vi "Export File - Tx Packet XML.vi"(4 "Tx Packet":T1 {"threadOptions"."pclDecimation" max=16 step=1; "threadOptions"."loopPeriod" max=16 step=1; "threadOptions"."targetPriority" min=-2 max=16 step=1; "threadOptions"."targetProcessor" min=-2 max=16 step=1; "Endianness" items=["big-endian"=0, "little-endian"=2]}, 6 "RootNode":refnum<k24>, 8 "error in (no error)":errorcluster, 9 "Tx Packet Header Data":T13, 11 "XmlDocument in":refnum<k24>) -> (0 "error out":errorcluster, 3 "XmlDocument out":refnum<k24>)   [LabVIEW 2019, in "UDP-Custom-Device System Explorer.lvlib"]
uses:
  UDP-Custom-Device System Explorer.lvlib
  System.Xml
  Types/XML - New/ImpExp - Packet Headers.ctl
  Types/XML - New/ImpExp - Tx Packet Data.ctl
  <vilib>/NI VeriStand/Custom Device API/Custom Device Item Info.ctl
  Shared/Types/Shared - Channel Data Type.ctl
  Shared/Types/Shared - Buffered.PacketInfo.ctl
  Shared/Types/Shared - Pointer Encoding.ctl
  Shared/Types/Shared - Receive Buffer Options.ctl
  Shared/Types/Shared - Transmit Buffer Options.ctl
  Shared/Types/Shared - Transmit Flag Options.ctl
  Shared/Types/Shared - Transmit Echo Options.ctl
  Types/Threading/Thread Configuration.ctl
  Types/Threading/Thread Sync Reference.ctl
  Shared/Types/Shared - Thread Management.ctl
  Shared/UDP-Custom-Device Shared.lvlib
  <vilib>/NI VeriStand/Custom Device API/Custom Device API.lvlib
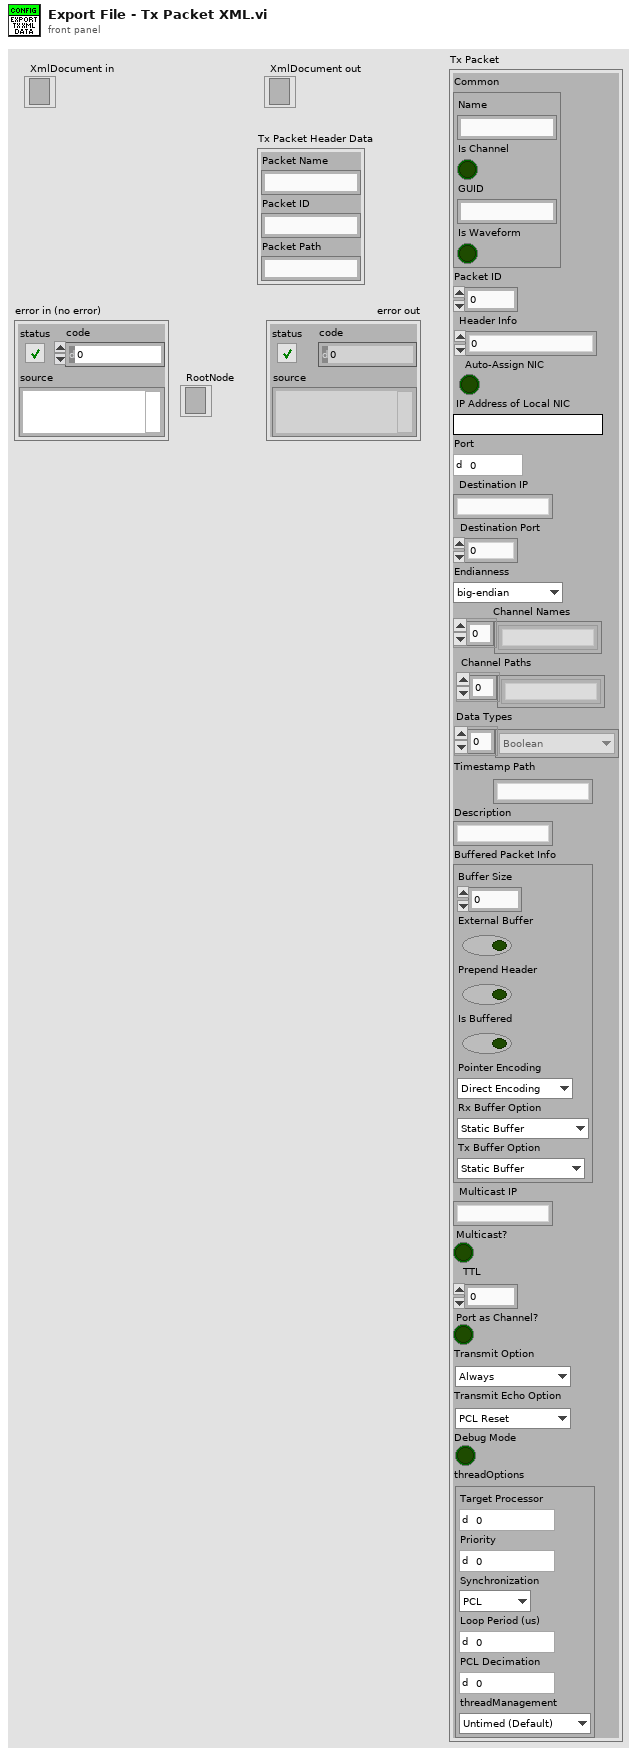
[diagram p1: front panel]
types:
  T1 = typedef "UDP-Custom-Device System Explorer.lvlib/ImpExp - Tx Packet Data.ctl" = cluster{"Common":T2, "Packet ID":i32, "Header Info":u32, "Auto-Assign NIC":bool, "IP Address of Local NIC":string, "Port":u16, "Destination IP":string, "Destination Port":u16, "Endianness":u16, "Channel Names":string[], "Channel Paths":string[], "Data Types":T3[], "Timestamp Path":string, "Description":string, "Buffered Packet Info":T4, "Multicast IP":string, "Multicast?":bool, "TTL":u16, "Port as Channel?":bool, "Transmit Option":T8, "Transmit Echo Option":T9, "Debug Mode":bool, "threadOptions":T10}
  T2 = typedef "Custom Device API.lvlib/Custom Device Item Info.ctl" = cluster{"Name":string, "Is Channel":bool, "GUID":string, "Is Waveform":bool}
  T3 = typedef "UDP-Custom-Device Shared.lvlib/Shared - Channel Data Type.ctl" = enum16{"Boolean", "Single", "Double", "I8", "I16", "I32", "I64", "U8", "U16", "U32", "U64"}
  T4 = typedef "UDP-Custom-Device Shared.lvlib/Shared - Buffered.PacketInfo.ctl" = cluster{"Buffer Size":i32, "External Buffer":bool, "Prepend Header":bool, "Is Buffered":bool, "Pointer Encoding":T5, "Rx Buffer Option":T6, "Tx Buffer Option":T7}
  T5 = typedef "UDP-Custom-Device Shared.lvlib/Shared - Pointer Encoding.ctl" = enum16{"Direct Encoding", "Conversion Encoding"}
  T6 = typedef "UDP-Custom-Device Shared.lvlib/Shared - Receive Buffer Options.ctl" = enum16{"Static Buffer", "Circular Buffer", "Circular Buffer + Size", "Internal Cache", "Internal Cache + Size", "Ping Pong", "Ping Pong + Size"}
  T7 = typedef "UDP-Custom-Device Shared.lvlib/Shared - Transmit Buffer Options.ctl" = enum16{"Static Buffer", "FIFO Buffer", "FIFO Buffer + Port"}
  T8 = typedef "UDP-Custom-Device Shared.lvlib/Shared - Transmit Flag Options.ctl" = enum16{"Always", "One-Shot", "Toggle"}
  T9 = typedef "UDP-Custom-Device Shared.lvlib/Shared - Transmit Echo Options.ctl" = enum16{"PCL Reset", "Counter", "Mirror"}
  T10 = typedef "UDP-Custom-Device System Explorer.lvlib/Thread Configuration.ctl" = cluster{"targetProcessor":i8, "targetPriority":i16, "Synchronization":T11, "loopPeriod":u32, "pclDecimation":u16, "threadManagement":T12}
  T11 = typedef "UDP-Custom-Device System Explorer.lvlib/Thread Sync Reference.ctl" = enum16{"PCL", "Async"}
  T12 = typedef "UDP-Custom-Device Shared.lvlib/Shared - Thread Management.ctl" = enum16{"Untimed (Default)", "Timed (High Priority)"}
  T13 = typedef "UDP-Custom-Device System Explorer.lvlib/ImpExp - Packet Headers.ctl" = cluster{"Packet Name":string, "Packet ID":string, "Packet Path":string}
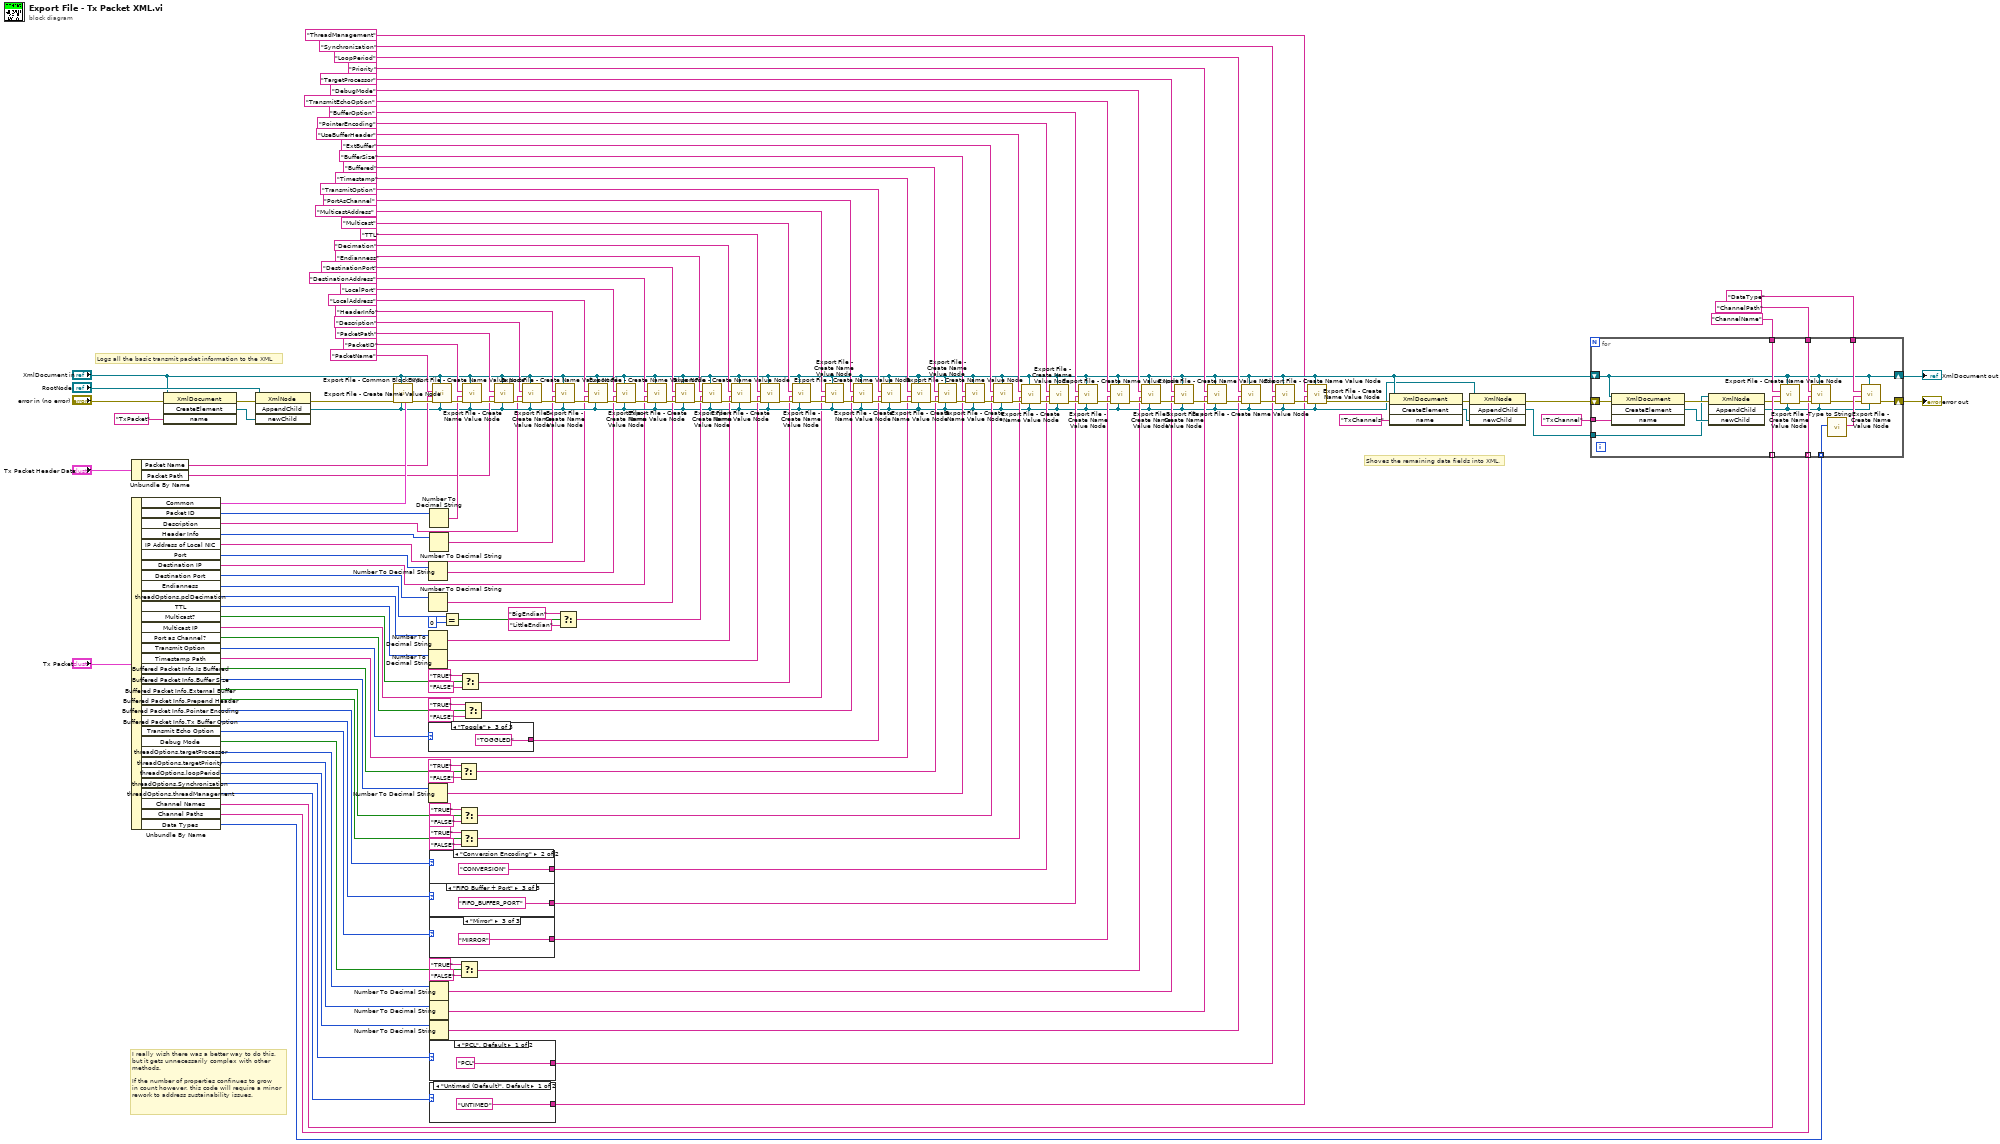
[diagram p0: block diagram]
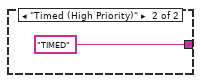
[diagram p2: hidden frame]
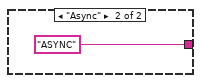
[diagram p3: hidden frame]
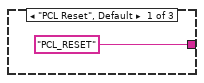
[diagram p4: hidden frame]
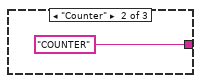
[diagram p5: hidden frame]
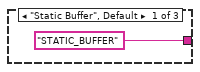
[diagram p6: hidden frame]
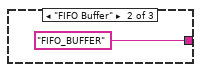
[diagram p7: hidden frame]
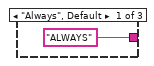
[diagram p8: hidden frame]
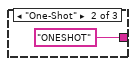
[diagram p9: hidden frame]
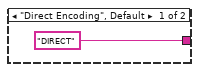
[diagram p10: hidden frame]
diagram:
  # "I really wish there was a better way to do this,\nbut it gets unnecessarily complex with other\nmethods.\n\nIf the number of properties confinues to grow\nin count however, this code will require a minor\nrework to address sustainability issues."
  # "Shoves the remaining data fields into XML."
  # "Logs all the basic transmit packet information to the XML"
  n1 = Unbundle By Name("Tx Packet") -> ("Common"=w149:T2, "Packet ID"=w140:i32, "Description"=w25:string, "Header Info"=w115:u32, "IP Address of Local NIC"=w24:string, "Port"=w112:u16, "Destination IP"=w23:string, "Destination Port"=w110:u16, "Endianness"=w103:u16, "threadOptions.pclDecimation"=w108:u16, "TTL"=w22:u16, "Multicast?"=w21:bool, "Multicast IP"=w20:string, "Port as Channel?"=w19:bool, "Transmit Option"=w18:T8, "Timestamp Path"=w17:string, "Buffered Packet Info.Is Buffered"=w16:bool, "Buffered Packet Info.Buffer Size"=w15:i32, "Buffered Packet Info.External Buffer"=w14:bool, "Buffered Packet Info.Prepend Header"=w13:bool, "Buffered Packet Info.Pointer Encoding"=w12:T5, "Buffered Packet Info.Tx Buffer Option"=w11:T7, "Transmit Echo Option"=w10:T9, "Debug Mode"=w9:bool, "threadOptions.targetProcessor"=w8:i8, "threadOptions.targetPriority"=w7:i16, "threadOptions.loopPeriod"=w6:u32, "threadOptions.Synchronization"=w5:T11, "threadOptions.threadManagement"=w4:T12, "Channel Names"=w3:string[], "Channel Paths"=w2:string[], "Data Types"=w1:T3[])
  n2 = Unbundle By Name("Tx Packet Header Data") -> ("Packet Name"=w139:string, "Packet Path"=w137:string)
  n3 = invoke class="XmlDocument" method="CreateElement"(reference="XmlDocument in", error in="error in (no error)", "name"="TxPacket" ("Tag Name")) -> (error out=w153:errorcluster, "CreateElement"=w154:refnum<k24>)  [unwired: 1 in, 2 out]
  n4 = invoke class="XmlNode" method="AppendChild"(reference="RootNode", error in=w153, "newChild"=w154) -> (error out=w152:errorcluster, "AppendChild"=w28:refnum<k24>)  [unwired: 1 in, 2 out]
  n5 = call "Export File - Common Block XML.vi"("Common"=w149, "RootNode in"=w28, "XmlDocument in"="XmlDocument in", "error in (no error)"=w152) -> ("error out"=w142:errorcluster)  [unwired: 7 in]
  n6 = Number To Decimal String(number=w112) -> (decimal integer string=w111:string)  [unwired: 1 in]
  n7 = Number To Decimal String(number=w110) -> (decimal integer string=w109:string)  [unwired: 1 in]
  n8 = Number To Decimal String(number=w108) -> (decimal integer string=w107:string)  [unwired: 1 in]
  n9 = Number To Decimal String(number=w22) -> (decimal integer string=w68:string)  [unwired: 1 in]
  n10 = case shown="\"Toggle\"" w18 {
    tunnel: ["ALWAYS" "ONESHOT" "TOGGLED"] -> w55
    frame "Always", Default {
    }
    frame "One-Shot" {
    }
    frame "Toggle" {
    }
  }
  n11 = Number To Decimal String(number=w15) -> (decimal integer string=w94:string)  [unwired: 1 in]
  n12 = Number To Decimal String(number=w140) -> (decimal integer string=w138:string)  [unwired: 1 in]
  n13 = Number To Decimal String(number=w115) -> (decimal integer string=w114:string)  [unwired: 1 in]
  n14 = case shown="\"Conversion Encoding\"" w12 {
    tunnel: ["DIRECT" "CONVERSION"] -> w64
    frame "Direct Encoding", Default {
    }
    frame "Conversion Encoding" {
    }
  }
  n15 = case shown="\"FIFO Buffer + Port\"" w11 {
    tunnel: ["STATIC_BUFFER" "FIFO_BUFFER" "FIFO_BUFFER_PORT"] -> w52
    frame "Static Buffer", Default {
    }
    frame "FIFO Buffer" {
    }
    frame "FIFO Buffer + Port" {
    }
  }
  n16 = case shown="\"Mirror\"" w10 {
    tunnel: ["PCL_RESET" "COUNTER" "MIRROR"] -> w49
    frame "PCL Reset", Default {
    }
    frame "Counter" {
    }
    frame "Mirror" {
    }
  }
  n17 = Number To Decimal String(number=w8) -> (decimal integer string=w35:string)  [unwired: 1 in]
  n18 = Number To Decimal String(number=w7) -> (decimal integer string=w34:string)  [unwired: 1 in]
  n19 = Number To Decimal String(number=w6) -> (decimal integer string=w33:string)  [unwired: 1 in]
  n20 = case shown="\"PCL\", Default" w5 {
    tunnel: ["PCL" "ASYNC"] -> w32
    frame "PCL", Default {
    }
    frame "Async" {
    }
  }
  n21 = case shown="\"Untimed (Default)\", Default" w4 {
    tunnel: ["UNTIMED" "TIMED"] -> w26
    frame "Untimed (Default)", Default {
    }
    frame "Timed (High Priority)" {
    }
  }
  n22 = call "Export File - Create Name Value Node.vi"("RootNode in"=w28, "XmlDocument in"="XmlDocument in", "error in (no error)"=w142, "Value"=w139, "Name"="PacketName" ("Tag Name")) -> ("error out"=w147:errorcluster)  [unwired: 6 in]
  n23 = Equal?(x=w103, y=u16 0) -> (x = y?=w102:bool)
  n24 = Select(t="TRUE", s=w16, f="FALSE") -> (s? t:f=w96:string)
  n25 = Select(t="TRUE", s=w14, f="FALSE") -> (s? t:f=w89:string)
  n26 = Select(t="TRUE", s=w13, f="FALSE") -> (s? t:f=w88:string)
  n27 = Select(t="TRUE", s=w9, f="FALSE") -> (s? t:f=w44:string)
  n28 = Select(t="TRUE", s=w21, f="FALSE") -> (s? t:f=w69:string)
  n29 = call "Export File - Create Name Value Node.vi"("RootNode in"=w28, "XmlDocument in"="XmlDocument in", "error in (no error)"=w147, "Value"=w138, "Name"="PacketID" ("Tag Name")) -> ("error out"=w146:errorcluster)  [unwired: 6 in]
  n30 = Select(t="TRUE", s=w19, f="FALSE") -> (s? t:f=w59:string)
  n31 = call "Export File - Create Name Value Node.vi"("RootNode in"=w28, "XmlDocument in"="XmlDocument in", "error in (no error)"=w146, "Value"=w137, "Name"="PacketPath" ("Tag Name")) -> ("error out"=w130:errorcluster)  [unwired: 6 in]
  n32 = call "Export File - Create Name Value Node.vi"("RootNode in"=w28, "XmlDocument in"="XmlDocument in", "error in (no error)"=w130, "Value"=w25, "Name"="Description" ("Tag Name")) -> ("error out"=w136:errorcluster)  [unwired: 6 in]
  n33 = call "Export File - Create Name Value Node.vi"("RootNode in"=w28, "XmlDocument in"="XmlDocument in", "error in (no error)"=w136, "Value"=w114, "Name"="HeaderInfo" ("Tag Name")) -> ("error out"=w113:errorcluster)  [unwired: 6 in]
  n34 = Select(t="BigEndian", s=w102, f="LittleEndian") -> (s? t:f=w101:string)
  n35 = call "Export File - Create Name Value Node.vi"("RootNode in"=w28, "XmlDocument in"="XmlDocument in", "error in (no error)"=w113, "Value"=w24, "Name"="LocalAddress" ("Tag Name")) -> ("error out"=w135:errorcluster)  [unwired: 6 in]
  n36 = call "Export File - Create Name Value Node.vi"("RootNode in"=w28, "XmlDocument in"="XmlDocument in", "error in (no error)"=w135, "Value"=w111, "Name"="LocalPort" ("Tag Name")) -> ("error out"=w134:errorcluster)  [unwired: 6 in]
  n37 = call "Export File - Create Name Value Node.vi"("RootNode in"=w28, "XmlDocument in"="XmlDocument in", "error in (no error)"=w134, "Value"=w23, "Name"="DestinationAddress" ("Tag Name")) -> ("error out"=w133:errorcluster)  [unwired: 6 in]
  n38 = call "Export File - Create Name Value Node.vi"("RootNode in"=w28, "XmlDocument in"="XmlDocument in", "error in (no error)"=w133, "Value"=w109, "Name"="DestinationPort" ("Tag Name")) -> ("error out"=w132:errorcluster)  [unwired: 6 in]
  n39 = call "Export File - Create Name Value Node.vi"("RootNode in"=w28, "XmlDocument in"="XmlDocument in", "error in (no error)"=w132, "Value"=w101, "Name"="Endianness" ("Tag Name")) -> ("error out"=w131:errorcluster)  [unwired: 6 in]
  n40 = call "Export File - Create Name Value Node.vi"("RootNode in"=w28, "XmlDocument in"="XmlDocument in", "error in (no error)"=w131, "Value"=w107, "Name"="Decimation" ("Tag Name")) -> ("error out"=w74:errorcluster)  [unwired: 6 in]
  n41 = call "Export File - Create Name Value Node.vi"("RootNode in"=w28, "XmlDocument in"="XmlDocument in", "error in (no error)"=w74, "Value"=w68, "Name"="TTL" ("Tag Name")) -> ("error out"=w76:errorcluster)  [unwired: 6 in]
  n42 = call "Export File - Create Name Value Node.vi"("RootNode in"=w28, "XmlDocument in"="XmlDocument in", "error in (no error)"=w76, "Value"=w69, "Name"="Multicast" ("Tag Name")) -> ("error out"=w75:errorcluster)  [unwired: 6 in]
  n43 = call "Export File - Create Name Value Node.vi"("RootNode in"=w28, "XmlDocument in"="XmlDocument in", "error in (no error)"=w75, "Value"=w20, "Name"="MulticastAddress" ("Tag Name")) -> ("error out"=w63:errorcluster)  [unwired: 6 in]
  n44 = call "Export File - Create Name Value Node.vi"("RootNode in"=w28, "XmlDocument in"="XmlDocument in", "error in (no error)"=w63, "Value"=w59, "Name"="PortAsChannel" ("Tag Name")) -> ("error out"=w58:errorcluster)  [unwired: 6 in]
  n45 = call "Export File - Create Name Value Node.vi"("RootNode in"=w28, "XmlDocument in"="XmlDocument in", "error in (no error)"=w58, "Value"=w55, "Name"="TransmitOption" ("Tag Name")) -> ("error out"=w57:errorcluster)  [unwired: 6 in]
  n46 = call "Export File - Create Name Value Node.vi"("RootNode in"=w28, "XmlDocument in"="XmlDocument in", "error in (no error)"=w57, "Value"=w17, "Name"="Timestamp" ("Tag Name")) -> ("error out"=w98:errorcluster)  [unwired: 6 in]
  n47 = call "Export File - Create Name Value Node.vi"("RootNode in"=w28, "XmlDocument in"="XmlDocument in", "error in (no error)"=w98, "Value"=w96, "Name"="Buffered" ("Tag Name")) -> ("error out"=w97:errorcluster)  [unwired: 6 in]
  n48 = call "Export File - Create Name Value Node.vi"("RootNode in"=w28, "XmlDocument in"="XmlDocument in", "error in (no error)"=w97, "Value"=w94, "Name"="BufferSize" ("Tag Name")) -> ("error out"=w119:errorcluster)  [unwired: 6 in]
  n49 = call "Export File - Create Name Value Node.vi"("RootNode in"=w28, "XmlDocument in"="XmlDocument in", "error in (no error)"=w119, "Value"=w89, "Name"="ExtBuffer" ("Tag Name")) -> ("error out"=w118:errorcluster)  [unwired: 6 in]
  n50 = call "Export File - Create Name Value Node.vi"("RootNode in"=w28, "XmlDocument in"="XmlDocument in", "error in (no error)"=w118, "Value"=w88, "Name"="UseBufferHeader" ("Tag Name")) -> ("error out"=w66:errorcluster)  [unwired: 6 in]
  n51 = call "Export File - Create Name Value Node.vi"("RootNode in"=w28, "XmlDocument in"="XmlDocument in", "error in (no error)"=w66, "Value"=w64, "Name"="PointerEncoding" ("Tag Name")) -> ("error out"=w54:errorcluster)  [unwired: 6 in]
  n52 = call "Export File - Create Name Value Node.vi"("RootNode in"=w28, "XmlDocument in"="XmlDocument in", "error in (no error)"=w54, "Value"=w52, "Name"="BufferOption" ("Tag Name")) -> ("error out"=w51:errorcluster)  [unwired: 6 in]
  n53 = call "Export File - Create Name Value Node.vi"("RootNode in"=w28, "XmlDocument in"="XmlDocument in", "error in (no error)"=w51, "Value"=w49, "Name"="TransmitEchoOption" ("Tag Name")) -> ("error out"=w46:errorcluster)  [unwired: 6 in]
  n54 = call "Export File - Create Name Value Node.vi"("RootNode in"=w28, "XmlDocument in"="XmlDocument in", "error in (no error)"=w46, "Value"=w44, "Name"="DebugMode" ("Tag Name")) -> ("error out"=w40:errorcluster)  [unwired: 6 in]
  n55 = call "Export File - Create Name Value Node.vi"("RootNode in"=w28, "XmlDocument in"="XmlDocument in", "error in (no error)"=w40, "Value"=w35, "Name"="TargetProcessor" ("Tag Name")) -> ("error out"=w41:errorcluster)  [unwired: 6 in]
  n56 = call "Export File - Create Name Value Node.vi"("RootNode in"=w28, "XmlDocument in"="XmlDocument in", "error in (no error)"=w41, "Value"=w34, "Name"="Priority" ("Tag Name")) -> ("error out"=w43:errorcluster)  [unwired: 6 in]
  n57 = call "Export File - Create Name Value Node.vi"("RootNode in"=w28, "XmlDocument in"="XmlDocument in", "error in (no error)"=w43, "Value"=w33, "Name"="LoopPeriod" ("Tag Name")) -> ("error out"=w42:errorcluster)  [unwired: 6 in]
  n58 = call "Export File - Create Name Value Node.vi"("RootNode in"=w28, "XmlDocument in"="XmlDocument in", "error in (no error)"=w42, "Value"=w32, "Name"="Synchronization" ("Tag Name")) -> ("error out"=w31:errorcluster)  [unwired: 6 in]
  n59 = call "Export File - Create Name Value Node.vi"("RootNode in"=w28, "XmlDocument in"="XmlDocument in", "error in (no error)"=w31, "Value"=w26, "Name"="ThreadManagement" ("Tag Name")) -> ("error out"=w30:errorcluster)  [unwired: 6 in]
  n60 = invoke class="XmlDocument" method="CreateElement"(reference="XmlDocument in", error in=w30, "name"="TxChannels" ("Tag Name")) -> (error out=w85:errorcluster, "CreateElement"=w87:refnum<k24>)  [unwired: 1 in, 2 out]
  n61 = invoke class="XmlNode" method="AppendChild"(reference=w28, error in=w85, "newChild"=w87) -> (error out=w84:errorcluster, "AppendChild"=w78:refnum<k24>)  [unwired: 1 in, 2 out]
  n62 = for {
    shift-right: [w188] -> w81
    shift-left: w84 -> [w175]
    shift-right: [w176] -> w80
    shift-left: "XmlDocument in" -> [w176]
    tunnel: "ChannelName" ("Tag Name") -> [w187]
    tunnel: "DataType" ("Tag Name") -> [w186]
    tunnel: w3 -> [w185] mode=indexing
    tunnel: w1 -> [w184] mode=indexing
    tunnel: "ChannelPath" ("Tag Name") -> [w180]
    tunnel: w2 -> [w179] mode=indexing
    tunnel: w78 -> [w173]
    tunnel: "TxChannel" ("Tag Name") -> [w172]
    n63 = invoke class="XmlDocument" method="CreateElement"(reference=w176, error in=w175, "name"=w172) -> (error out=w177:errorcluster, "CreateElement"=w178:refnum<k24>)  [unwired: 1 in, 2 out]
    n64 = invoke class="XmlNode" method="AppendChild"(reference=w173, error in=w177, "newChild"=w178) -> (error out=w174:errorcluster, "AppendChild"=w171:refnum<k24>)  [unwired: 1 in, 2 out]
    n65 = call "Export File - Create Name Value Node.vi"("RootNode in"=w171, "XmlDocument in"=w176, "error in (no error)"=w174, "Value"=w185, "Name"=w187) -> ("error out"=w182:errorcluster)  [unwired: 6 in]
    n66 = call "Export File - Create Name Value Node.vi"("RootNode in"=w171, "XmlDocument in"=w176, "error in (no error)"=w182, "Value"=w179, "Name"=w180) -> ("error out"=w181:errorcluster)  [unwired: 6 in]
    n67 = call "Type to String.vi"("Data Type"=w184) -> ("String Type"=w183:string)  [unwired: 10 in]
    n68 = call "Export File - Create Name Value Node.vi"("RootNode in"=w171, "XmlDocument in"=w176, "error in (no error)"=w181, "Value"=w183, "Name"=w186) -> ("error out"=w188:errorcluster)  [unwired: 6 in]
  }
  "error out" <- w81
  "XmlDocument out" <- w80
